vi "tests12.vi"   [LabVIEW 2012]
uses:
  <vilib>/NXT/Subs/MotorOutput.ctl
  <vilib>/NXT/Dual Mode Library/Display/drawNumber_float.vi
  <vilib>/NXT/Dual Mode Library/Waits/Wait_Num.vi
types:
  T1 = typedef "MotorOutput.ctl" = u8
  T2 = typedef "LVHSConnector.ctl" = cluster{"Hardware":string, "Flattened String":string}
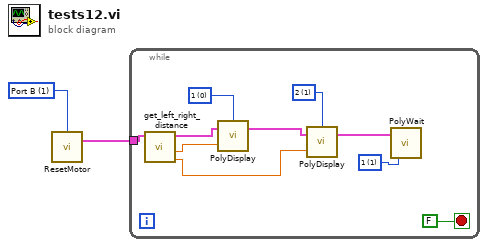
[diagram p0: block diagram]
diagram:
  w2 = T1 1 items=["Port A"=0, "Port B"=1, "Port C"=2, "Ports A & B"=4, "Ports A & C"=5, "Ports B & C"=6, "All Ports"=3] ("Output Port (All Ports)")
  n1 = call <vilib>:"ResetMotor.vi"("Port (All Ports)"=w2) -> ("NXT"=w1:T2)  [unwired: 3 in]
  n2 = while {
    tunnel: w1 -> [w12]
    stop <- FALSE stop-if-true
    w4 = i16 1 items=["1", "1", "3", "4", "5", "6", "7", "8"] ("Line")
    w10 = i16 1 items=["1", "2", "3", "4", "5", "6", "7", "8"] ("Line")
    w11 = i16 0 items=["1", "2", "3", "4", "5", "6", "7", "8"] ("Line")
    n3 = call "get_left_right_distance.vi"("NXT"=w12) -> ("right distance"=w6:dbl, "left distance"=w7:dbl, "NXT 2"=w9:T2)  [unwired: 8 in]
    n4 = call-poly <vilib>:"PolyDisplay.vi"("number"=w7, "NXT"=w9, "Line"=w11) -> ("NXT"=w8:T2)  [unwired: 1 in]
    n5 = call-poly <vilib>:"PolyDisplay.vi"("number"=w6, "NXT"=w8, "Line"=w10) -> ("NXT"=w5:T2)  [unwired: 1 in]
    n6 = call-poly <vilib>:"PolyWait.vi"("Time (1 sec)"=w4, "NXT"=w5) -> ()  [unwired: 2 in, 1 out]
  }
